vi "WD_Cylinder_Up.vi"(7 "位置(記錄用)":string="790", 8 "error in (no error)":errorcluster, 9 "禁止覆蓋":bool, 10 "Workplace_id":i16, 11 "DBLink":string) -> (2 "當前資料":cluster{"條碼R":string, "條碼L":string}, 3 "DBLink ref":string)   [LabVIEW 2019]
panel:
  # "此id位置為汽缸剛頂起，需搬移資料至此欄位"
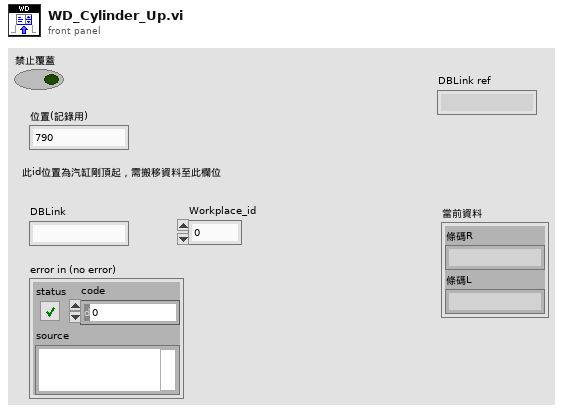
[diagram p1: front panel]
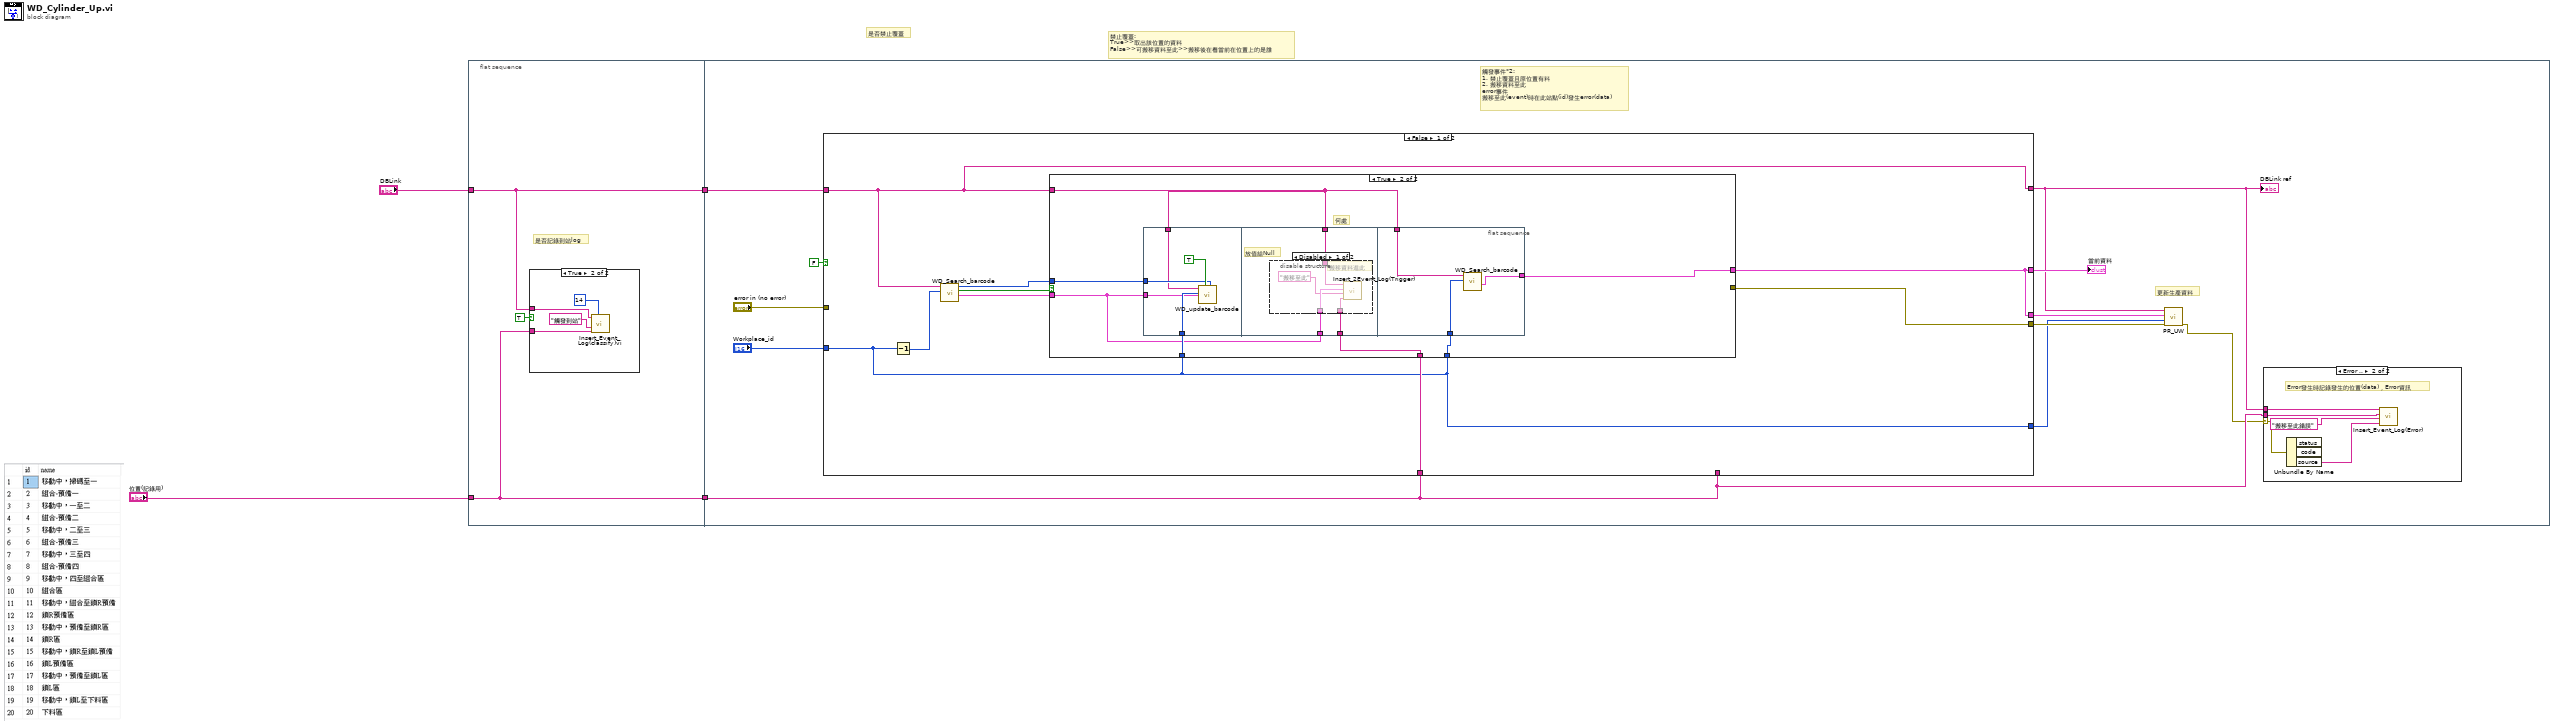
[diagram p0: block diagram]
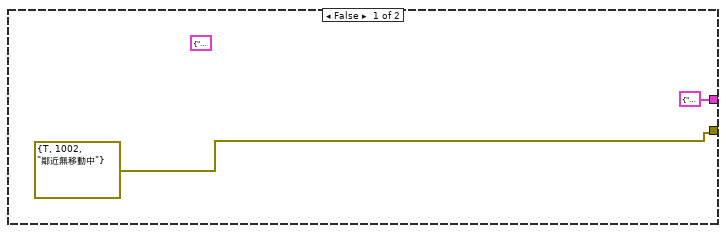
[diagram p3: hidden frame]
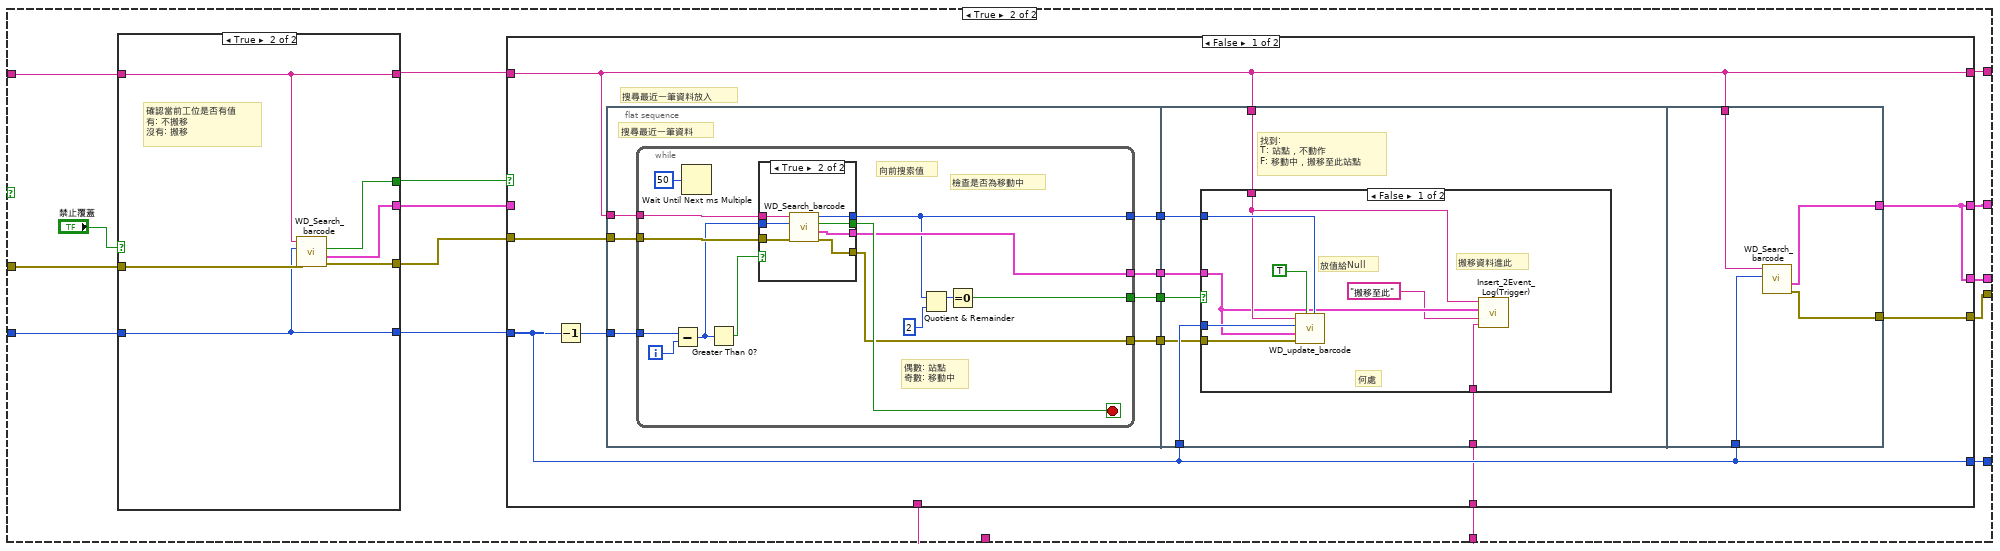
[diagram p5: hidden frame]
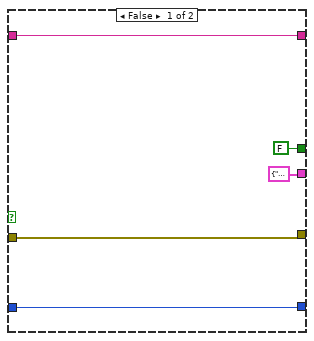
[diagram p6: hidden frame]
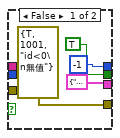
[diagram p7: hidden frame]
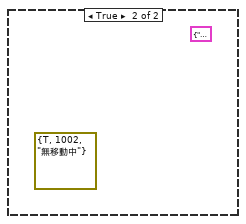
[diagram p8: hidden frame]
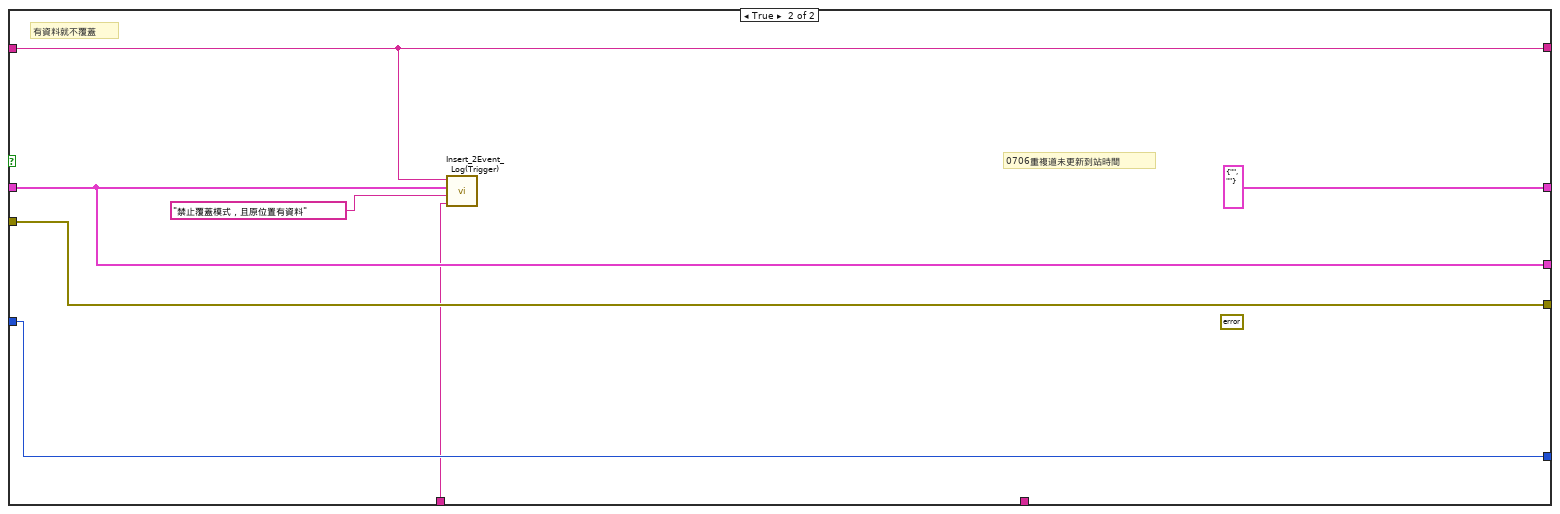
[diagram p9: hidden frame]
diagram:
  # "是否禁止覆蓋"
  # "禁止覆蓋:\nTrue>>取出該位置的資料\nFalse>>可搬移資料至此>>搬移後在看當前在位置上的是誰"
  n1 = flat-sequence {
    tunnel: "位置(記錄用)" -> [w7]
    tunnel: "DBLink" -> [w6]
    tunnel: [w6] -> w2
    tunnel: [w7] -> w1
    tunnel: w2 -> [w22]
    tunnel: w1 -> [w13]
    frame #0 {
      # "是否記錄到站log"
      n2 = case shown="True" TRUE {
        tunnel: w7 -> [_ w11]
        tunnel: w6 -> [_ w10]
        frame False {
        }
        frame True {
          n3 = call "Insert_Event_Log(classify)vi.vi"("classify"=i16 14, "data"=w11, "message"="觸發到站", "DBlink"=w10) -> ()  [unwired: 7 in, 1 out]
        }
      }
    }
    frame #1 {
      # "觸發事件*2: \n1. 禁止覆蓋且原位置有料\n2. 搬移資料至此\nerror事件\n搬移至此(event)時在此站點(id)發生error(data)"
      # "更新生產資料"
      n4 = case shown="False" FALSE {
        tunnel: w22 -> [w23 w70]
        tunnel: "error in (no error)" -> [_ w69]
        tunnel: "Workplace_id" -> [w25 w68]
        tunnel: [w26 w61] -> w19
        tunnel: [w25 w60] -> w18
        tunnel: [w24 w59] -> w17
        tunnel: [w24 w58] -> w16
        tunnel: [w23 w57] -> w15
        tunnel: w13 -> [_ w56]
        tunnel: w13 -> [w27 _]
        frame False {
          n5 = Decrement(x=w25) -> (x-1=w31:i16)
          n6 = call "WD_Search_barcode.vi"("workplace_name_id"=w31, "DBlink"=w23) -> ("workplace_data"=w29:cluster{"條碼R":string, "條碼L":string}, "找到"=w30:bool, "取得ID"=w28:i16)  [unwired: 6 in, 1 out]
          n7 = case shown="True" w30 {
            tunnel: w23 -> [_ w35]
            tunnel: w25 -> [_ w40]
            tunnel: w29 -> [_ w37]
            tunnel: w28 -> [_ w39]
            tunnel: w27 -> [_ w38]
            tunnel: w25 -> [_ w36]
            tunnel: [cluster{"條碼R":string, "條碼L":string} {"條碼R"="", "條碼L"=""} ("workplace_data") w34] -> w24
            tunnel: [errorcluster {"status"=TRUE, "code"=1002, "source"="鄰近無移動中"} ("error constant") _] -> w26
            frame False {
              (unwired) cluster{"條碼R":string, "條碼L":string} {"條碼R"="", "條碼L"=""} ("workplace_data")
            }
            frame True {
              # "何處"
              n8 = flat-sequence {
                tunnel: w40 -> [w44]
                tunnel: w39 -> [w43]
                tunnel: w37 -> [w42]
                tunnel: w35 -> [w41]
                tunnel: w38 -> [w48]
                tunnel: w35 -> [w47]
                tunnel: w37 -> [w46]
                tunnel: w36 -> [w55]
                tunnel: w35 -> [w54]
                tunnel: [w53] -> w34
                frame #0 {
                  n9 = call "WD_update_barcode.vi"("NULL: workplace_id"=w43, "Set null"=TRUE, "Workplace data"=w42, "workplace_id"=w44, "DBlink"=w41) -> ()  [unwired: 7 in]
                }
                frame #1 {
                  # "放值給Null"
                  n10 = disable-structure shown="Disabled" {
                    disable-tunnel: w48 -> [w52 _]
                    disable-tunnel: w47 -> [w51 _]
                    disable-tunnel: w46 -> [w50 _]
                    frame Disabled {
                      # "搬移資料進此"
                      n11 = call "Insert_2Event_Log(Trigger).vi"("data"=w52, "message"="搬移至此", "output cluster"=w50, "DBlink"=w51) -> ()  [unwired: 8 in]
                    }
                    frame Enabled {
                    }
                  }
                }
                frame #2 {
                  n12 = call "WD_Search_barcode.vi"("workplace_name_id"=w55, "DBlink"=w54) -> ("workplace_data"=w53:cluster{"條碼R":string, "條碼L":string})  [unwired: 6 in, 3 out]
                }
              }
            }
          }
        }
        frame True {
          n13 = case shown="True" "禁止覆蓋" {
            tunnel: w70 -> [w72 w79]
            tunnel: w69 -> [w75 w81]
            tunnel: w68 -> [w74 w80]
            tunnel: [w74 w80] -> w66
            tunnel: [w72 w79] -> w65
            tunnel: [FALSE ("找到") w78] -> w64
            tunnel: [w75 w77] -> w63
            tunnel: [cluster{"條碼R":string, "條碼L":string} {"條碼R"="", "條碼L"=""} ("workplace_data") w76] -> w62
            frame False {
            }
            frame True {
              # "確認當前工位是否有值\n有: 不搬移\n沒有: 搬移"
              n14 = call "WD_Search_barcode.vi"("error in (no error)"=w81, "workplace_name_id"=w80, "DBlink"=w79) -> ("error out"=w77:errorcluster, "workplace_data"=w76:cluster{"條碼R":string, "條碼L":string}, "找到"=w78:bool)  [unwired: 5 in, 1 out]
            }
          }
          n15 = case shown="False" w64 {
            tunnel: w63 -> [w92 w150]
            tunnel: w66 -> [w86 w149]
            tunnel: w65 -> [w88 w147]
            tunnel: [w87 w150] -> w61
            tunnel: [w83 cluster{"條碼R":string, "條碼L":string} {"條碼R"="", "條碼L"=""} ("workplace_data")] -> w59
            tunnel: w62 -> [_ w146]
            tunnel: [w88 w147] -> w57
            tunnel: [w86 w149] -> w60
            tunnel: [w83 w146] -> w58
            tunnel: w56 -> [w82 _]
            tunnel: w56 -> [_ w144]
            frame False {
              # "搜尋最近一筆資料放入"
              n16 = Decrement(x=w86) -> (x-1=w91:i16)
              n17 = flat-sequence {
                tunnel: w88 -> [w99]
                tunnel: w92 -> [w98]
                tunnel: w91 -> [w97]
                tunnel: [w96] -> w90
                tunnel: [w95] -> w89
                tunnel: [w94] -> w85
                tunnel: [w93] -> w84
                tunnel: w90 -> [w131]
                tunnel: w88 -> [w130]
                tunnel: w86 -> [w129]
                tunnel: w89 -> [w128]
                tunnel: w85 -> [w127]
                tunnel: w84 -> [w126]
                tunnel: w82 -> [w125]
                tunnel: w88 -> [w143]
                tunnel: w86 -> [w142]
                tunnel: [w141] -> w83
                tunnel: [w140] -> w87
                frame #0 {
                  # "搜尋最近一筆資料"
                  n18 = while {
                    tunnel: w99 -> [w113]
                    tunnel: w98 -> [w111]
                    tunnel: w97 -> [w108]
                    tunnel: [w105] -> w96
                    tunnel: [w104] -> w95
                    tunnel: [w101] -> w94
                    tunnel: [w100] -> w93
                    i -> [w112]
                    stop <- w107 stop-if-true
                    # "偶數: 站點\n奇數: 移動中"
                    # "檢查是否為移動中"
                    # "向前搜索值"
                    n19 = Subtract(x=w108, y=w112) -> (x-y=w106:i32)
                    n20 = Wait Until Next ms Multiple(millisecond multiple=u32 50) -> ()  [unwired: 1 out]
                    n21 = Greater Than 0?(x=w106) -> (x > 0?=w110:bool)
                    n22 = case shown="True" w110 {
                      tunnel: w113 -> [_ w124]
                      tunnel: w111 -> [_ w123]
                      tunnel: [errorcluster {"status"=TRUE, "code"=1001, "source"="id<0\n無值"} ("error out") w122] -> w104
                      tunnel: w106 -> [_ w121]
                      tunnel: [TRUE ("找到") w120] -> w107
                      tunnel: [i16 -1 ("取得ID") w119] -> w100
                      tunnel: [cluster{"條碼A":string, "條碼B":string} {"條碼A"="", "條碼B"=""} ("workplace_data") w118] -> w105
                      frame False {
                      }
                      frame True {
                        n23 = call "WD_Search_barcode.vi"("error in (no error)"=w123, "workplace_name_id"=w121, "DBlink"=w124) -> ("error out"=w122:errorcluster, "workplace_data"=w118:cluster{"條碼R":string, "條碼L":string}, "找到"=w120:bool, "取得ID"=w119:i16)  [unwired: 5 in]
                      }
                    }
                    n24 = Quotient & Remainder(x=w100, y=2) -> (x-y*floor(x/y)=w103:i32)  [unwired: 1 out]
                    n25 = Equal To 0?(x=w103) -> (x = 0?=w101:bool)
                  }
                }
                frame #1 {
                  # "找到: \nT: 站點，不動作\nF: 移動中，搬移至此站點"
                  n26 = case shown="False" w127 {
                    tunnel: w131 -> [w134 _]
                    tunnel: w130 -> [w135 _]
                    tunnel: w129 -> [w138 _]
                    tunnel: w128 -> [w137 _]
                    tunnel: w126 -> [w136 _]
                    tunnel: w125 -> [w132 _]
                    frame False {
                      # "何處"
                      # "搬移資料進此"
                      # "放值給Null"
                      n27 = call "WD_update_barcode.vi"("NULL: workplace_id"=w136, "Set null"=TRUE, "error in (no error)"=w137, "Workplace data"=w134, "workplace_id"=w138, "DBlink"=w135) -> ()  [unwired: 6 in]
                      n28 = call "Insert_2Event_Log(Trigger).vi"("data"=w132, "message"="搬移至此", "output cluster"=w134, "DBlink"=w135) -> ()  [unwired: 8 in]
                    }
                    frame True {
                      (unwired) errorcluster {"status"=TRUE, "code"=1002, "source"="無移動中"} ("error constant")
                      (unwired) cluster{"條碼R":string, "條碼L":string} {"條碼R"="", "條碼L"=""} ("workplace_data")
                    }
                  }
                }
                frame #2 {
                  n29 = call "WD_Search_barcode.vi"("workplace_name_id"=w142, "DBlink"=w143) -> ("error out"=w140:errorcluster, "workplace_data"=w141:cluster{"條碼R":string, "條碼L":string})  [unwired: 6 in, 2 out]
                }
              }
            }
            frame True {
              (unwired) errorcluster {"status"=FALSE, "code"=0, "source"=""} ("error constant")
              # "0706重複道未更新到站時間"
              # "有資料就不覆蓋"
              n30 = call "Insert_2Event_Log(Trigger).vi"("data"=w144, "message"="禁止覆蓋模式，且原位置有資料", "output cluster"=w146, "DBlink"=w147) -> ()  [unwired: 8 in]
            }
          }
        }
      }
      "當前資料" <- w17
      "DBLink ref" <- w15
      n31 = call "PR_UW .vi"("error in (no error)"=w19, "[workplace_id]"=w18, "當前工位資料"=w16, "DBlink"=w15) -> ("error out"=w12:errorcluster)  [unwired: 7 in]
      n32 = case shown="Error .." w12 {
        selector: w12 -> [_ w152]
        tunnel: w15 -> [_ w155]
        tunnel: w13 -> [_ w153]
        frame No Error {
        }
        frame Error {
          # "Error發生時記錄發生的位置(data)，Error資訊"
          n33 = Unbundle By Name(w152) -> ("source"=w151:string)  [unwired: 2 out]
          n34 = call "Insert_Event_Log(Error).vi"("data"=w151, "message"="搬移至此錯誤", "id"=w153, "DBlink"=w155) -> ()  [unwired: 8 in]
        }
      }
    }
  }
